vi "WarpAffineGreyscale.vi"(4 "Border Colour (Default: 0)":u8, 5 "Boarder Type (Default: DEFAULT)":T2=enum."DEFAULT", 6 "Required Destination Size":T4, 7 "Interpolation Mode (Default: CUBIC)":T3=enum."CUBIC", 8 "error in (no error)":errorcluster, 9 "2x3 Affine Matrix":T1, 10 "Greyscale Destination Image":refnum<data-value>, 11 "Greyscale Source Image":refnum<data-value>) -> (0 "error out":errorcluster, 3 "Greyscale Destination Image (duplicate)":refnum<data-value>)   [LabVIEW 2020, in "g_ar_toolkit.image.lvlib"]
uses:
  g_ar_toolkit.image.lvlib
  g_ar_toolkit.common/Image Size (Integer).ctl
  Interpolation Mode.ctl
  Border Type.ctl
  <vilib>/Analysis/Matrix/Datatypes/RealMatrix.ctl
  b7e6b07f-7daf-4958-9fc0-179f1836a141.vi/0c263cf4-9042-4d44-b92e-dafa676e1650.vi
  <vilib>/Utility/error.llb/Error Cluster From Error Code.vi
  b7e6b07f-7daf-4958-9fc0-179f1836a141.vi
  g_ar_toolkit.common/g_ar_toolkit_common.lvlib
  <vilib>/Analysis/Matrix/NI_Matrix.lvlib
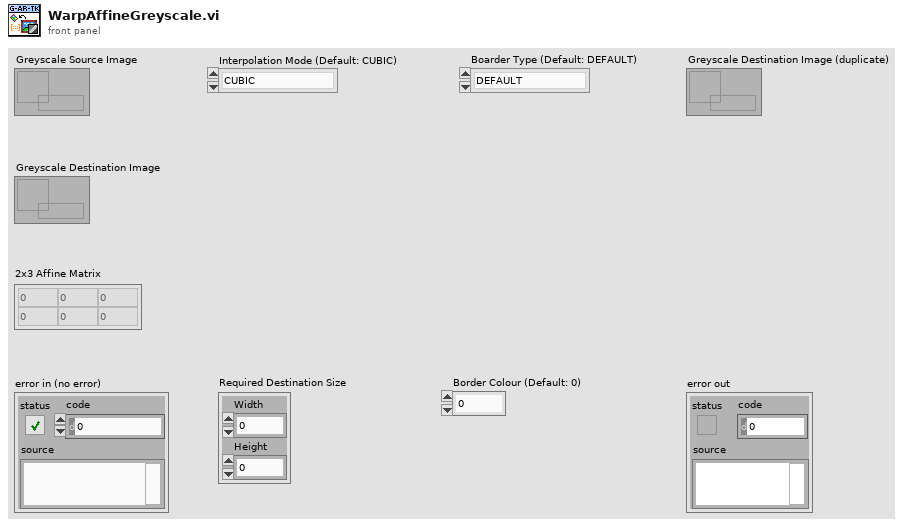
[diagram p1: front panel]
types:
  T1 = typedef "NI_Matrix.lvlib/RealMatrix.ctl" = dbl[][]
  T2 = typedef "g_ar_toolkit.image.lvlib/Border Type.ctl" = enum8{"CONSTANT", "REPLICATE", "REFLECT", "WRAP", "TRANSPARENT", "DEFAULT", "ISOLATED"}
  T3 = typedef "g_ar_toolkit.image.lvlib/Interpolation Mode.ctl" = enum8{"NEAREST", "LINEAR", "CUBIC", "AREA", "LANCZOS", "LINEAR_EXACT", "NEAREST_EXACT", "MAX"}
  T4 = typedef "g_ar_toolkit_common.lvlib/Image Size (Integer).ctl" = cluster{"Width":u16, "Height":u16}
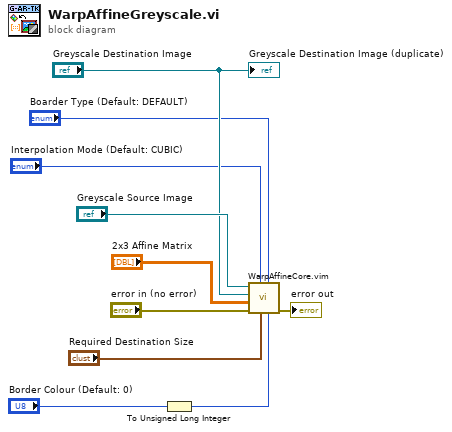
[diagram p0: block diagram]
diagram:
  n1 = To Unsigned Long Integer(number="Border Colour (Default: 0)") -> (unsigned 32bit integer=w1:u32)
  n2 = call "WarpAffineCore.vim"("Border Colour"=w1, "Boarder Type"="Boarder Type (Default: DEFAULT)", "Destination Size"="Required Destination Size", "Interpolation Mode"="Interpolation Mode (Default: CUBIC)", "error in (no error)"="error in (no error)", "Affine"="2x3 Affine Matrix", "Dst"="Greyscale Destination Image", "Src"="Greyscale Source Image") -> ("error out"=→"error out":errorcluster)  [unwired: 3 in]
  "Greyscale Destination Image (duplicate)" <- "Greyscale Destination Image"
